vi "LEER PUERTO SERIAL S ENTERO v2.vi"(4 "caracter terminador":string, 5 "read buffer":string, 6 "buffer de datos":i32[](array[numeric]), 7 "buffer in":string) -> (0 "indicador de llegada de datos":bool, 2 "salida datos numericos":i32[](array[numeric]), 3 "buffer out":string)   [LabVIEW 2017]
doc: "Codigo para arduino:\n\n Serial.println(Xint);\n Serial.println(Yint);\n Serial.println(\"P\");\n\nDonde P es el caracter de terminacion de cadena\nXint y Yint son datos de tipo entero"
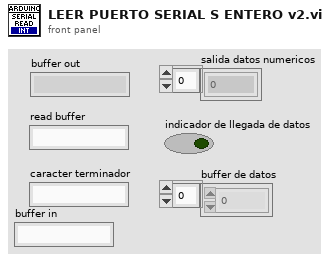
[diagram p1: front panel]
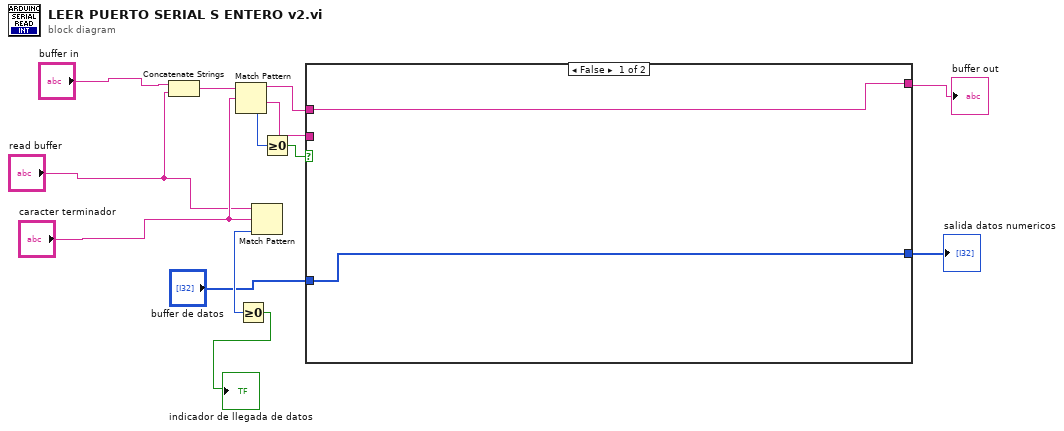
[diagram p0: block diagram]
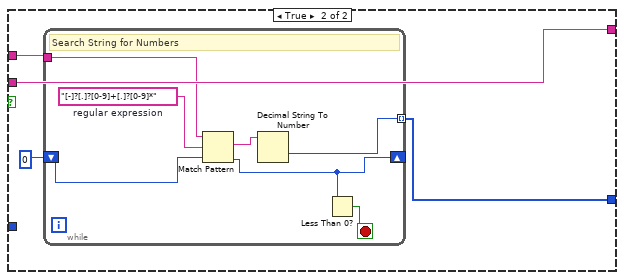
[diagram p2: hidden frame]
diagram:
  n1 = Concatenate Strings("buffer in", "read buffer") -> (w6:string)
  n2 = Match Pattern(string=w6, regular expression="caracter terminador") -> (before substring=w5:string, after substring=w7:string, offset past match=w9:i32)  [unwired: 1 in, 1 out]
  n3 = Match Pattern(string="read buffer", regular expression="caracter terminador") -> (offset past match=w4:i32)  [unwired: 1 in, 3 out]
  n4 = Greater Or Equal To 0?(x=w4) -> (x >= 0?=→"indicador de llegada de datos":bool)
  n5 = Greater Or Equal To 0?(x=w9) -> (x >= 0?=w8:bool)
  n6 = case shown="False" w8 {
    tunnel: w7 -> [_ w19]
    tunnel: [w15 w19] -> w10
    tunnel: w5 -> [w15 w17]
    tunnel: "buffer de datos" -> [w14 _]
    tunnel: [w14 w16] -> w1
    frame False {
    }
    frame True {
      n7 = while {
        shift-left: 0 -> [w24]
        shift-right: [w22] -> _
        tunnel: [w26] -> w16 mode=indexing
        tunnel: w17 -> [w20]
        stop <- w25 stop-if-true
        w21 = "[-]?[.]?[0-9]+[.]?[0-9]*"  # regular expression
        # "Search String for Numbers"
        n8 = Match Pattern(string=w20, regular expression=w21, offset (0)=w24) -> (match substring=w23:string, offset past match=w22:i32)  [unwired: 2 out]
        n9 = Decimal String To Number(string=w23) -> (number=w26:i32)  [unwired: 2 in, 1 out]
        n10 = Less Than 0?(x=w22) -> (x < 0?=w25:bool)
      }
    }
  }
  "buffer out" <- w10
  "salida datos numericos" <- w1
